vi "coordinate_structure2array_vector.vi"(0 "Fiducial_Pos_structure":T1) -> (1 "Current_Instrument_pos":dbl[](array[numeric]), 2 "Reference_Instrument_pos":dbl[](array[numeric]))   [LabVIEW 2011]
doc: "This routine takes the paired fiducial structure and converts it to two arrays (i.e. vectors)"
uses:
  Fiducial_pair.ctl
panel:
  # "Fiducial Location Pair"
  # "Current Instrument Fiducial Location"
  # "Reference Instrument Fiducial Location"
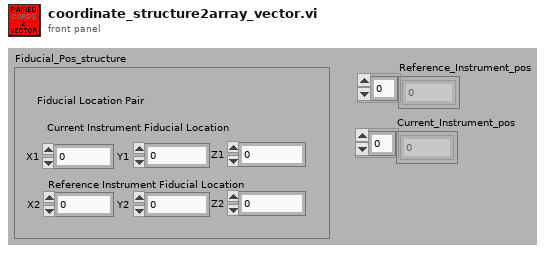
[diagram p1: front panel]
types:
  T1 = typedef "Fiducial_pair.ctl" = cluster{"X1":dbl, "X2":dbl, "Y1":dbl, "Y2":dbl, "Z1":dbl, "Z2":dbl}
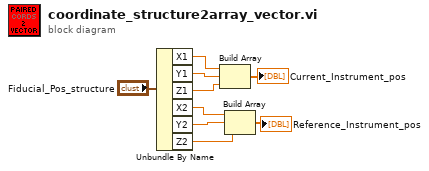
[diagram p0: block diagram]
diagram:
  n1 = Unbundle By Name("Fiducial_Pos_structure") -> ("X1"=w3:dbl, "Y1"=w2:dbl, "Z1"=w1:dbl, "X2"=w4:dbl, "Y2"=w5:dbl, "Z2"=w6:dbl)
  n2 = Build Array(w3, w2, w1) -> (→"Current_Instrument_pos":dbl[])
  n3 = Build Array(w4, w5, w6) -> (→"Reference_Instrument_pos":dbl[])
